vi "ReadAppDataFromFile.vi"(8 "ErrorArray In":errorcluster[](array[cluster]), 11 "TestFileRef In":T2) -> (0 "ErrorArray Out":errorcluster[](array[cluster]), 2 "clAppData":T1, 3 "TestFileRef out":T2)   [LabVIEW 2017, in "Framework.lvlib"]
uses:
  Framework.lvlib
  <vilib>/Utility/config.llb/Config Data RefNum.ctl
  <vilib>/Utility/error.llb/Error Cluster From Error Code.vi
  <vilib>/ErrorRing/Error Ring.xnode
  <userlib>/NIST/NISTErrorLib/NISTErrorLib.lvlib
  <vilib>/Utility/config.llb/NI_LVConfig.lvlib
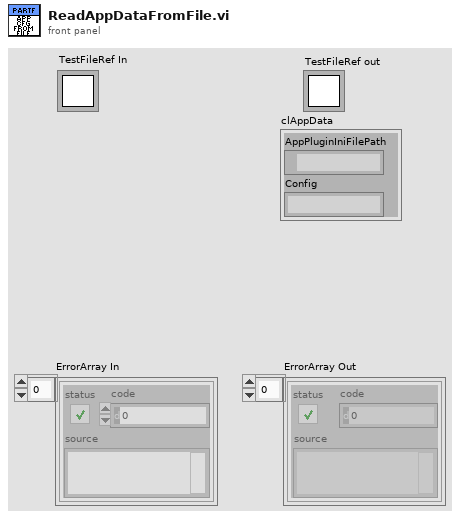
[diagram p1: front panel]
types:
  T1 = cluster{"AppPluginIniFilePath":path, "Config":string}
  T2 = typedef "NI_LVConfig.lvlib/Config Data RefNum.ctl" = refnum<k1>
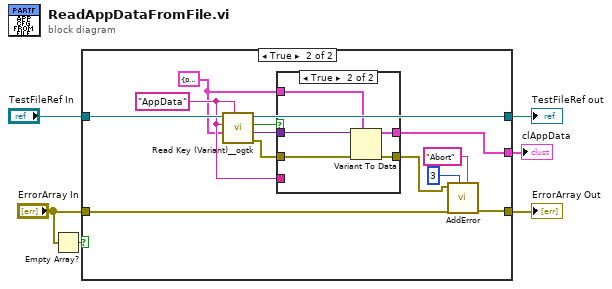
[diagram p0: block diagram]
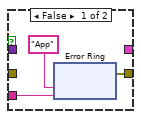
[diagram p3: hidden frame]
diagram:
  n1 = Empty Array?(array="ErrorArray In") -> (empty?=w5:bool)
  n2 = case shown="True" w5 {
    tunnel: "ErrorArray In" -> [w8 w16]
    tunnel: [w8 w15] -> w4
    tunnel: [w7 w18] -> w2
    tunnel: "TestFileRef In" -> [w7 w21]
    tunnel: [_ w17] -> w1
    frame False {
    }
    frame True {
      w9 = T1 {"AppPluginIniFilePath"=path "", "Config"=""} ("clAppData")
      w10 = "AppData" ("section")
      n3 = call <userlib>:"Read Key (Variant)__ogtk.vi"("section"=w10, "type"=w9, "key (optional)"=w10, "refnum"=w21) -> ("error out"=w19:errorcluster, "key-value"=w20:variant, "found?"=w11:bool, "refnum out"=w18:T2)  [unwired: 4 in]
      n4 = case shown="True" w11 {
        tunnel: w20 -> [_ w37]
        tunnel: w19 -> [_ w36]
        tunnel: [_ w35] -> w17
        tunnel: [w24 w34] -> w12
        tunnel: w10 -> [w22 _]
        tunnel: w9 -> [_ w33]
        frame False {
          n5 = xnode "Error Ring"("parameter 0"="App", "parameter 1"=w22) -> ("error out"=w24:errorcluster)
        }
        frame True {
          n6 = Variant To Data(error in=w36, type=w33, Variant=w37) -> (data=w35:T1, error out=w34:errorcluster)
        }
      }
      n7 = call <userlib>:"AddError.vi"("Severity"="Abort", "Priority"=u8 3, "ErrorArray"=w16, "error in (no error)"=w12) -> ("ErrorArray"=w15:errorcluster[])  [unwired: 6 in, 1 out]
    }
  }
  "ErrorArray Out" <- w4
  "TestFileRef out" <- w2
  "clAppData" <- w1
